vi "DataToDB.vi"(8 "error in":errorcluster, 9 "all string":string="'TBOX','1805','34002001180314080000000014728956','08CAG2018031400000019','2018-07-10 10:16:30',@b", 10 "Procedure name":string, 11 "DSN name":string) -> (0 "error out":errorcluster, 1 "Certid":string, 2 "TUID":string, 3 "ReportStrA":string)   [LabVIEW 2013]
uses:
  <vilib>/addons/database/Connection.llb/DB Tools Open Connec (String).vi
  <vilib>/addons/database/Connection.llb/Conn Execute.vi
  <vilib>/addons/database/Recordset.llb/Rec Fetch Recordset Data (R).vi
  <vilib>/addons/database/Recordset.llb/Rec Destroy - Connection.vi
  <vilib>/addons/database/NI_Database_API.lvlib
panel:
  out "连接的字符串":string="prc_writeTuidCertid('TBOX','1805','34002001180314080000000014728956','08CAG2018031400000019','2018-07-10 10:16:30',@b)"
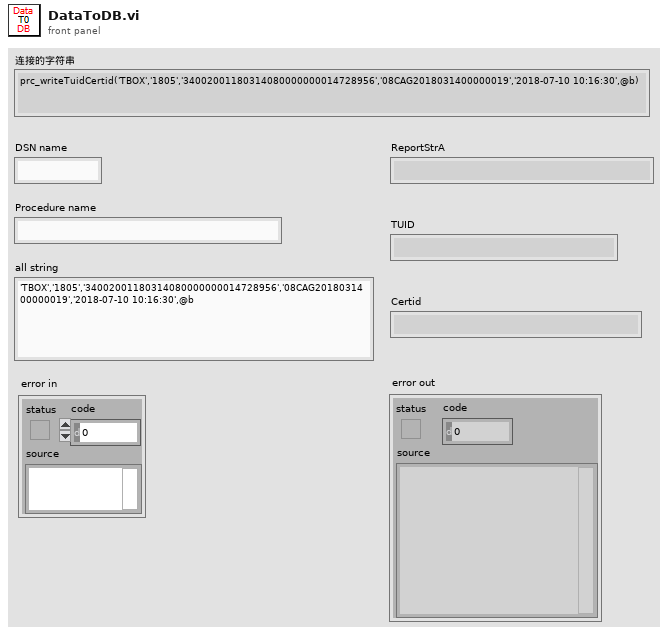
[diagram p1: front panel]
types:
  T1 = typedef "NI_Database_API.lvlib/Conn ObjectReference.ctl" = refnum<k1>
  T2 = typedef "NI_Database_API.lvlib/Rec ObjectReference.ctl" = refnum<k1>
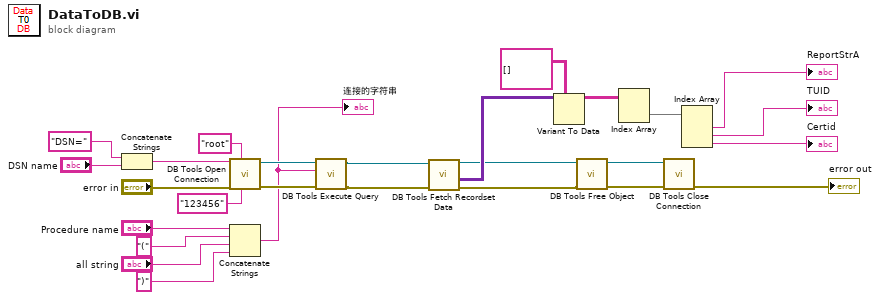
[diagram p0: block diagram]
diagram:
  n1 = Concatenate Strings("DSN=", "DSN name") -> (w17:string)
  n2 = call-poly <vilib>:"DB Tools Open Connection.vi"("password"="123456" ("userID"), "userID"="root", "error in (no error)"="error in", "connection information"=w17) -> ("error out"=w27:errorcluster, "connection reference"=w26:T1)  [unwired: 4 in]
  n3 = Concatenate Strings("Procedure name", "(", "all string", ")") -> (w22:string)
  "连接的字符串" <- w22
  n4 = call-poly <vilib>:"DB Tools Execute Query.vi"("error in (no error)"=w27, "SQL query"=w22, "connection reference"=w26) -> ("error out"=w10:errorcluster, "recordset reference"=w11:T2)  [unwired: 5 in]
  n5 = call-poly <vilib>:"DB Tools Fetch Recordset Data.vi"("error in (no error)"=w10, "recordset reference"=w11) -> ("error out"=w8:errorcluster, "recordset data"=w13:variant[][], "recordset reference out"=w9:T2)  [unwired: 3 in]
  n6 = Variant To Data(type=string[][] [], Variant=w13) -> (data=w1:string[][])  [unwired: 1 in, 1 out]
  n7 = call-poly <vilib>:"DB Tools Free Object.vi"("error in (no error)"=w8, "recordset reference"=w9) -> ("error out"=w24:errorcluster, "connection reference"=w25:T1)  [unwired: 8 in]
  n8 = Index Array(array=w1) -> (element=w7:string[])  [unwired: 2 in]
  n9 = call <vilib>:"DB Tools Close Connection.vi"("error in (no error)"=w24, "connection reference"=w25) -> ("error out"=→"error out":errorcluster)  [unwired: 5 in]
  n10 = Index Array(array=w7) -> (element #1=→"ReportStrA":string, element #2=→"TUID":string, element #3=→"Certid":string)  [unwired: 3 in]
